vi "setup_lc_jy.vi"(4 "yw":string, 5 "zc_luodi_num":string, 6 "didian":string, 7 "jsren":string, 8 "shuoming":string, 9 "yongtu":string="借用", 10 "id":string, 11 "zhriqi":string) -> (2 "error":errorcluster)   [LabVIEW 2017, in "Lib_code.lvlib"]
uses:
  Lib_code.lvlib
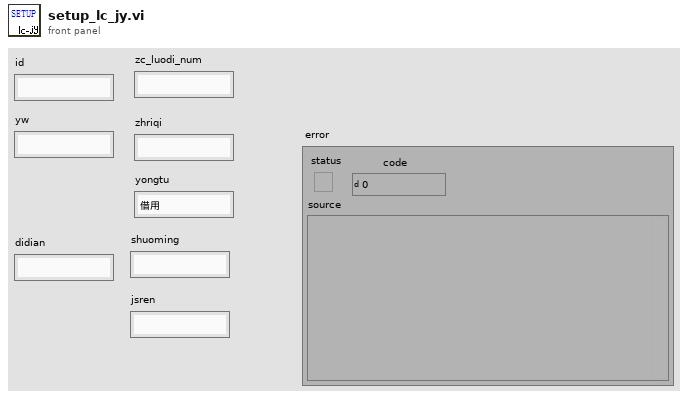
[diagram p1: front panel]
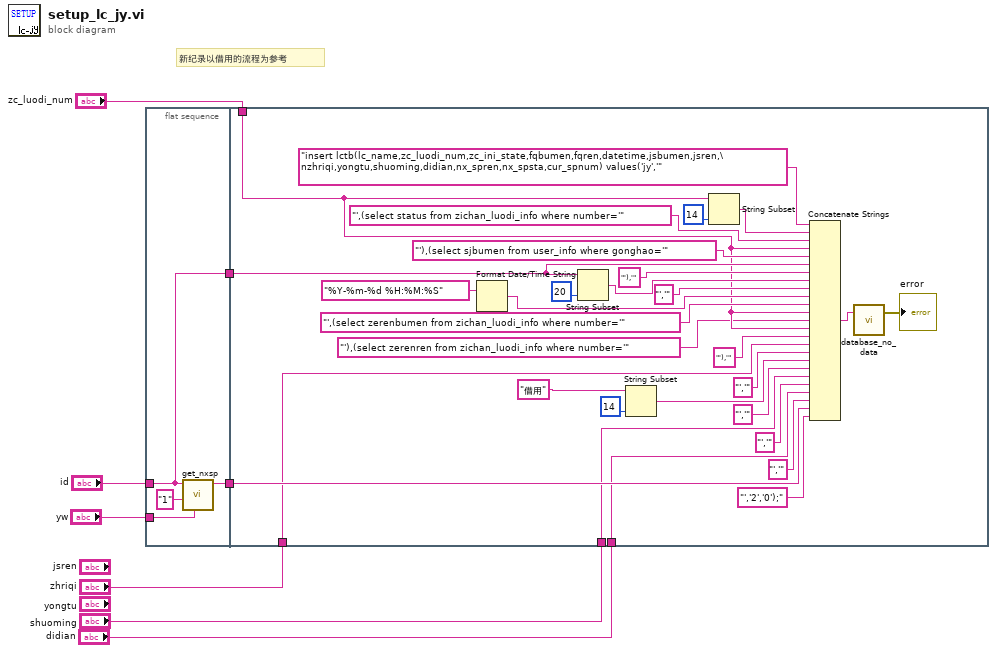
[diagram p0: block diagram]
diagram:
  # "新纪录以借用的流程为参考"
  n1 = flat-sequence {
    tunnel: [w12] -> w4
    tunnel: [w11] -> w3
    tunnel: "yw" -> [w10]
    tunnel: "id" -> [w11]
    tunnel: w4 -> [w34]
    tunnel: w3 -> [w28]
    tunnel: "zc_luodi_num" -> [w14]
    tunnel: "shuoming" -> [w23]
    tunnel: "zhriqi" -> [w26]
    tunnel: "didian" -> [w21]
    frame #0 {
      n2 = call "get_nxsp.vi"("yw"=w10, "Cur_state"="1", "fqren"=w11) -> ("sp_gonghao"=w12:string)  [unwired: 6 in, 2 out]
    }
    frame #1 {
      n3 = Format Date/Time String(time format string (%c)="%Y-%m-%d %H:%M:%S" ("时间格式字符串(%c)")) -> (date/time string=w18:string)  [unwired: 2 in]
      n4 = String Subset(string=w28, length (rest)=20 ("长度（剩余）")) -> (substring=w19:string)  [unwired: 1 in]
      n5 = String Subset(string="借用" ("字符串"), length (rest)=14 ("长度（剩余）")) -> (substring=w30:string)  [unwired: 1 in]
      n6 = String Subset(string=w14, length (rest)=14 ("长度（剩余）")) -> (substring=w40:string)  [unwired: 1 in]
      n7 = Concatenate Strings("insert lctb(lc_name,zc_luodi_num,zc_ini_state,fqbumen,fqren,datetime,jsbumen,jsren,\nzhriqi,yongtu,shuoming,didian,nx_spren,nx_spsta,cur_spnum) values('jy','" ("格式字符串"), w40, "',(select status from zichan_luodi_info where number='" ("字符串"), w14, "'),(select sjbumen from user_info where gonghao='" ("字符串"), w28, "'),'" ("字符串"), w19, "','" ("字符串"), w18, "',(select zerenbumen from zichan_luodi_info where number='" ("字符串"), w14, "'),(select zerenren from zichan_luodi_info where number='" ("字符串"), w14, "'),'" ("字符串"), w26, "','" ("字符串"), w30, "','" ("字符串"), w23, "','" ("字符串"), w21, "','" ("字符串"), w34, "','2','0');" ("字符串")) -> (w25:string)
      n8 = call "database_no_data.vi"("input"=w25) -> ("error"=→"error":errorcluster)  [unwired: 2 in]
    }
  }
